vi "Program_Pulse.vi"(8 "error in (no error)":errorcluster, 10 "Numeric":dbl, 11 "VISA Refnum in":refnum<visa-resource-name>) -> ()   [LabVIEW 2019]
uses:
  Viejos/Alfredo LABVIEW/Set-up verificador ASICs/Lib Agilent 81160A/Agilent 81150/Agilent 81150.lvlib
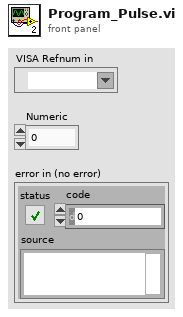
[diagram p1: front panel]
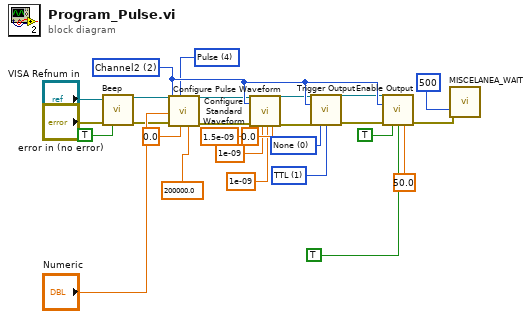
[diagram p0: block diagram]
diagram:
  w19 = u16 1 items=["ECL", "TTL"] ("Trigger Level Sync (0: ECL)")
  w18 = u16 0 items=["AB"=3, "B"=2, "A"=1, "None"=0] ("Trigger Sync Out (1: A)")
  w20 = u16 2 items=["Channel1"=1, "Channel2"=2] ("Channel (1: Channel1)")
  w11 = u16 4 items=["Sine", "Square", "Ramp Up", "Ramp Down", "Pulse", "Noise", "DC"] ("Waveform (0: Sine)")
  n1 = call "Beep.vi"("VISA resource name"="VISA Refnum in", "error in (no error)"="error in (no error)", "Beep (T: ON)"=TRUE) -> ("VISA resource name out"=w3:refnum<visa-resource-name>, "error out"=w4:errorcluster)  [unwired: 11 in]
  n2 = call "Configure Standard Waveform.vi"("Frequency (1000.0 Hz)"=200000.0, "DC Offset (0.0 Volts)"=0.0, "Waveform (0: Sine)"=w11, "error in (no error)"=w4, "Amplitude (1.0 Vpp)"="Numeric", "Channel (1: Channel1)"=w20, "VISA resource name"=w3) -> ("error out"=w9:errorcluster, "VISA resource name out"=w10:refnum<visa-resource-name>)  [unwired: 3 in]
  n3 = call "Configure Pulse Waveform.vi"("VISA resource name"=w10, "Channel (1: Channel1)"=w20, "error in (no error)"=w9, "Width (1.5E-9 Sec)"=1.5e-09, "Leading Edge Time\n(1.0E-9 Sec)"=1e-09 ("Leading Edge Time\n(1.0E-9 Sec)"), "Trailing Edge Time\n(1.0E-9 Sec)"=1e-09 ("Trailing Edge Time\n(1.0E-9 Sec)"), "Delay\n(0.0 Seconds)"=0.0 ("Delay\n(0.0 Seconds)")) -> ("VISA resource name out"=w8:refnum<visa-resource-name>, "error out"=w7:errorcluster)  [unwired: 11 in]
  n4 = call "Trigger Output.vi"("VISA resource name"=w8, "Channel (1: Channel1)"=w20, "error in (no error)"=w7, "Trigger Sync Out (1: A)"=w18, "Trigger Level Sync (0: ECL)"=w19) -> ("VISA resource name out"=w6:refnum<visa-resource-name>, "error out"=w5:errorcluster)  [unwired: 9 in]
  n5 = call "Enable Output.vi"("VISA resource name"=w6, "Channel (1: Channel1)"=w20, "error in (no error)"=w5, "Enable Output (T: Enable)"=TRUE, "Enable Output Complement (T: Enable)"=TRUE, "Load (50 Ohm)"=50.0) -> ("error out"=w2:errorcluster)  [unwired: 8 in, 1 out]
  n6 = call "MISCELANEA_WAIT.vi"("ms wait IN"=u32 500, "Error IN"=w2) -> ()  [unwired: 16 in, 2 out]
